vi "CalcMat.vi"(8 "error in (no error)":errorcluster, 11 "MultiBandState in":refnum<class "MultiBandState.lvclass">) -> (0 "error out":errorcluster, 3 "MultiBandState out":refnum<class "MultiBandState.lvclass">)   [LabVIEW 2018, in "Functions.lvlib" / "MultiBandState.lvclass"]
uses:
  MultiBandState.lvclass
  MultiBandState.lvclass/MultiBandState.ctl
  <vilib>/Analysis/Matrix/Datatypes/RealMatrix.ctl
  Accessors/Read MultiBand.vi
  Accessors/Read SampleRate.vi
  Accessors/Read MultiBandConfig.vi
  Accessors/Write MultiBand.vi
  <vilib>/Analysis/Matrix/Numeric/Conversions/Array To Matrix - RA2.vi
  <vilib>/Analysis/Matrix/NI_Matrix.lvlib
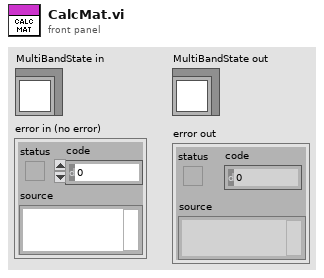
[diagram p1: front panel]
types:
  T1 = typedef "NI_Matrix.lvlib/RealMatrix.ctl" = dbl[][]
  T2 = cluster{"Handle":string, "Size":i32, "Gain":dbl, "Offset":dbl, "A":T1, "B":T1, "C":T1, "D":T1, "X":T1, "Waveform":waveform(dbl)}[]
  T3 = typedef "Functions.lvlib/MultiBandState.lvclass/clMultiBandConfig.ctl" = cluster{"Count":i32, "MultiBandConfig":T4[]}
  T4 = typedef "Functions.lvlib/MultiBandState.lvclass/MultiBandConfig.ctl" = cluster{"Handle":string, "Type":enum16{"Multiband", "Amplitude Modulation", "Phase Modulation", "Combined Modulation"}, "Freq":dbl[], "Index":dbl[], "Phase":dbl[][], "Damping":dbl[]}
  T5 = cluster{"Handle":string, "Size":i32, "Gain":dbl, "Offset":dbl, "A":T1, "B":T1, "C":T1, "D":T1, "X":T1, "Waveform":waveform(dbl)}
  T6 = enum16{"Multiband", "Amplitude Modulation", "Phase Modulation", "Combined Modulation"}
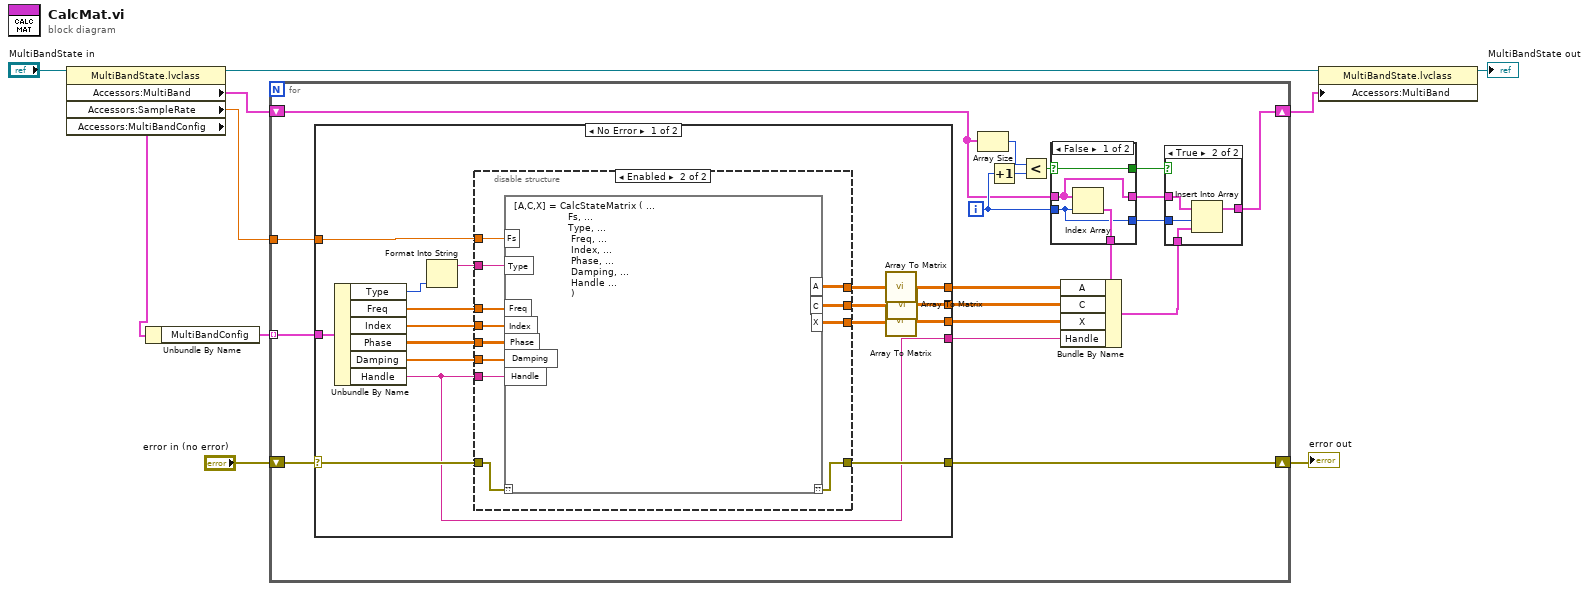
[diagram p0: block diagram]
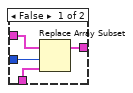
[diagram p2: hidden frame]
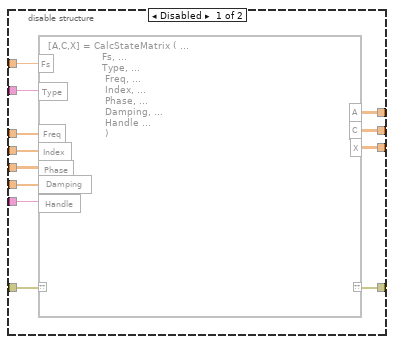
[diagram p3: hidden frame]
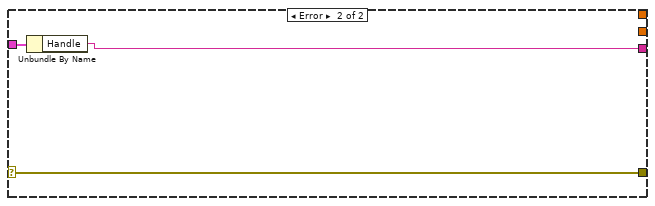
[diagram p4: hidden frame]
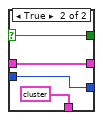
[diagram p5: hidden frame]
diagram:
  n1 = property class="MultiBandState.lvclass"(reference="MultiBandState in") -> (reference out=w5:refnum<class "MultiBandState.lvclass">, "Accessors:MultiBand"=w8:T2, "Accessors:SampleRate"=w9:dbl, "Accessors:MultiBandConfig"=w1:T3)  [unwired: 1 in, 1 out]
  n2 = Unbundle By Name(w1) -> ("MultiBandConfig"=w2:T4[])
  n3 = for {
    tunnel: w2 -> [w29] mode=indexing
    tunnel: w9 -> [w27]
    shift-right: [w12] -> w4
    shift-left: w8 -> [w16]
    shift-right: [w26] -> w3
    shift-left: "error in (no error)" -> [w28]
    i -> [w20]
    n4 = case shown="No Error" w28 {
      selector: w28 -> [w54 w79]
      tunnel: w29 -> [w52 w81]
      tunnel: w27 -> [w53 _]
      tunnel: [w44 _] -> w21
      tunnel: [w43 _] -> w22
      tunnel: [w42 _] -> w23
      tunnel: [w41 w79] -> w26
      tunnel: [w39 w80] -> w24
      frame No Error {
        n5 = Unbundle By Name(w52) -> ("Type"=w51:T6, "Freq"=w49:dbl[], "Index"=w48:dbl[], "Phase"=w38:dbl[][], "Damping"=w40:dbl[], "Handle"=w39:string)
        n6 = Format Into String(w51) -> (resulting string=w50:string)  [unwired: 3 in, 1 out]
        n7 = disable-structure shown="Enabled" {
          disable-tunnel: w54 -> [w66 w68]
          disable-tunnel: w53 -> [w65 w78]
          disable-tunnel: w50 -> [w64 w77]
          disable-tunnel: w49 -> [w63 w76]
          disable-tunnel: w48 -> [w62 w75]
          disable-tunnel: [w61 w71] -> w47
          disable-tunnel: [w60 w70] -> w46
          disable-tunnel: [w59 w69] -> w45
          disable-tunnel: [w58 w67] -> w41
          disable-tunnel: w40 -> [w57 w73]
          disable-tunnel: w39 -> [w56 w72]
          disable-tunnel: w38 -> [w55 w74]
          frame Disabled {
            n8 = script code="[A,C,X] = CalcStateMatrix ( ...\n                  Fs, ...\n                  Type, ...\n                   Freq, ...\n                   Index, ...\n                   Phase, ...\n                   Damping, ...\n                   Handle ...\n                   )"("??"=w66, "Fs"=w65, "Type"=w64, "Handle"=w56, "Freq"=w63, "Index"=w62, "Phase"=w55, "Damping"=w57) -> ("??"=w58:errorcluster, "A"=w61:dbl[][], "C"=w60:dbl[][], "X"=w59:dbl[][])
          }
          frame Enabled {
            n9 = script code="[A,C,X] = CalcStateMatrix ( ...\n                  Fs, ...\n                  Type, ...\n                   Freq, ...\n                   Index, ...\n                   Phase, ...\n                   Damping, ...\n                   Handle ...\n                   )"("??"=w68, "Fs"=w78, "Type"=w77, "Freq"=w76, "Index"=w75, "Phase"=w74, "Damping"=w73, "Handle"=w72) -> ("??"=w67:errorcluster, "A"=w71:dbl[][], "C"=w70:dbl[][], "X"=w69:dbl[][])
          }
        }
        n10 = call-poly <vilib>:"Array To Matrix.vi"("Real 2D Array"=w47) -> ("Real Matrix"=w44:T1)
        n11 = call-poly <vilib>:"Array To Matrix.vi"("Real 2D Array"=w45) -> ("Real Matrix"=w42:T1)
        n12 = call-poly <vilib>:"Array To Matrix.vi"("Real 2D Array"=w46) -> ("Real Matrix"=w43:T1)
      }
      frame Error {
        n13 = Unbundle By Name(w81) -> ("Handle"=w80:string)
      }
    }
    n14 = Array Size(array=w16) -> (size(s)=w18:i32)
    n15 = Increment(x=w20) -> (x+1=w19:i32)
    n16 = Less?(x=w18, y=w19) -> (x < y?=w17:bool)
    n17 = case shown="False" w17 {
      selector: w17 -> [w84 w88]
      tunnel: [w85 T5 {"Handle"="", "Size"=0, "Gain"=0.0, "Offset"=0.0, "A"=[], "B"=[], "C"=[], "D"=[], "X"=[], "Waveform"={"t0"=timestamp(0 s since 1904-01-01), "dt"=1.0, "Y"=[]}} ("MultiBand")] -> w25
      tunnel: w16 -> [w82 w86]
      tunnel: w20 -> [w83 w87]
      tunnel: [w84 w88] -> w15
      tunnel: [w83 w87] -> w14
      tunnel: [w82 w86] -> w11
      frame False {
        n18 = Index Array(array=w82, index=w83) -> (element=w85:T5)
      }
      frame True {
      }
    }
    n19 = Bundle By Name(cluster=w25, "A"=w21, "C"=w22, "X"=w23, "Handle"=w24) -> (w13:T5)
    n20 = case shown="True" w15 {
      tunnel: w14 -> [w33 w37]
      tunnel: w13 -> [w32 w36]
      tunnel: [w31 w35] -> w12
      tunnel: w11 -> [w30 w34]
      frame False {
        n21 = Replace Array Subset(array=w30, new element=w32, index=w33) -> (w31:T2)
      }
      frame True {
        n22 = Insert Into Array(array=w34, index=w37, new element=w36) -> (w35:T2)
      }
    }
  }
  "error out" <- w3
  n23 = property class="MultiBandState.lvclass"(reference=w5, "Accessors:MultiBand"=w4) -> (reference out=→"MultiBandState out":refnum<class "MultiBandState.lvclass">)  [unwired: 1 in, 1 out]
